vi "菜单演示.vi"() -> ()   [LabVIEW 2017]
panel:
  in  "Open(O)...":bool
  in  "Option(O)..":bool
  in  "Exit(X)":bool
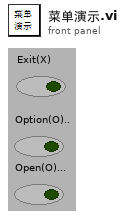
[diagram p1: front panel]
types:
  T1 = cluster{bool, "include Ctrl key?":bool, string}[]
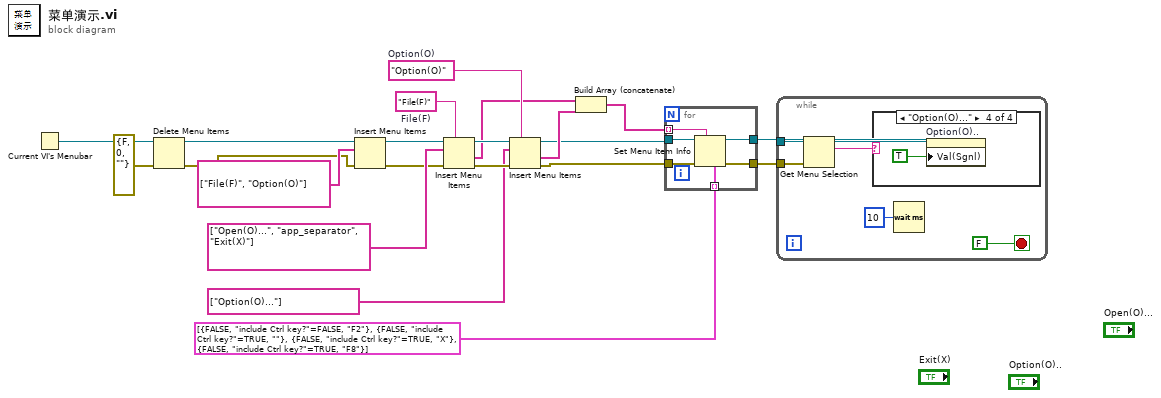
[diagram p0: block diagram]
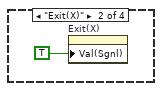
[diagram p3: hidden frame]
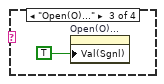
[diagram p4: hidden frame]
diagram:
  w14 = "Option(O)"  # Option(O)
  w15 = "File(F)"  # File(F)
  n1 = Current VI's Menubar() -> (w21:refnum<k9>)
  n2 = Delete Menu Items(6:errorcluster {"status"=FALSE, "code"=0, "source"=""} ("错误输入（无错误）"), 9:w21) -> (0:w9:errorcluster, 3:w20:refnum<k9>)  [unwired: 2 in]
  n3 = Insert Menu Items(6:w9, 8:string[] ["File(F)", "Option(O)"] ("项名称"), 9:w20) -> (0:w12:errorcluster, 3:w19:refnum<k9>)  [unwired: 3 in, 1 out]
  n4 = Insert Menu Items(5:w15, 6:w12, 8:string[] ["Open(O)...", "app_separator", "Exit(X)"] ("项名称"), 9:w19) -> (0:w11:errorcluster, 1:w6:string[], 3:w16:refnum<k9>)  [unwired: 2 in]
  n5 = Insert Menu Items(5:w14, 6:w11, 8:string[] ["Option(O)..."] ("项名称"), 9:w16) -> (0:w10:errorcluster, 1:w5:string[], 3:w3:refnum<k9>)  [unwired: 2 in]
  n6 = Build Array (concatenate)(w6, w5) -> (w13:string[])
  n7 = for {
    tunnel: w13 -> [w27] mode=indexing
    tunnel: [w26] -> w2
    tunnel: [w25] -> w1
    tunnel: w10 -> [w24]
    tunnel: T1 [{FALSE, "include Ctrl key?"=FALSE, "F2"}, {FALSE, "include Ctrl key?"=TRUE, ""}, {FALSE, "include Ctrl key?"=TRUE, "X"}, {FALSE, "include Ctrl key?"=TRUE, "F8"}] -> [w23] mode=indexing
    tunnel: w3 -> [w22]
    n8 = Set Menu Item Info(4:w23, 7:w27, 8:w24, 11:w22) -> (0:w25:errorcluster, 3:w26:refnum<k9>)  [unwired: 3 in]
  }
  n9 = while {
    tunnel: w2 -> [w31]
    tunnel: w1 -> [w28]
    stop <- FALSE stop-if-true
    n10 = Get Menu Selection(0:w31, 3:w28) -> (6:w30:string)  [unwired: 2 in, 4 out]
    n11 = case shown="\"Option(O)...\"" w30 {
      frame Default {
      }
      frame "Exit(X)" {
        n12 = property on="Exit(X)" class="Bool (严格)"("Val(Sgnl)"=TRUE ("值(信号)")) -> ()  [unwired: 2 in, 2 out]
      }
      frame "Open(O)..." {
        n13 = property on="Open(O)..." class="Bool (严格)"("Val(Sgnl)"=TRUE ("值(信号)")) -> ()  [unwired: 2 in, 2 out]
      }
      frame "Option(O)..." {
        n14 = property on="Option(O).." class="Bool (严格)"("Val(Sgnl)"=TRUE ("值(信号)")) -> ()  [unwired: 2 in, 2 out]
      }
    }
    n15 = Wait (ms)(milliseconds to wait=u32 10 ("等待时间（毫秒）")) -> ()  [unwired: 1 out]
  }
